vi "Keithley 6514 Buffer Config.vi"(0 "Resource In":refnum<visa-resource-name>, 1 "Check For SCPI Errors? (T)":bool=TRUE, 5 "Buffer Setup (Clear Buffer:0)":u16(ring) items=["Clear Buffer", "Configure Buffer"], 7 "Buffer Control (Never:0)":u16(ring) items=["Never", "Next"], 9 "Buffer Points (100)":i16=100 min=1 max=2500 step=1, 11 "error in (no error)":T1, 12 "TimeStamp Format (Absolute:0)":u16(ring) items=["Absolute", "Delta"], 13 "Reading Source\nfor Buffer (Sense (input):0)":u16(ring) items=["Sense (input)", "Calc1 (math)", "Calc2 (limits)"]) -> (4 "Resource Out (dupl)":refnum<visa-resource-name>, 15 "error out":T1)   [LabVIEW 2009, in "Keithley 6514 LV 2009.lvlib"]
doc: "This VI is used to configure the buffer for storing readings.\n\nDEFAULTS: GPIB Address = 14\n\nBuffer Setup:\n0 = Clear Buffer\n1 = Configure Buffer\n\nBuffer Control:\n0 = Never\n1 = Next\n\nBuffer Points:\n1 - 2500\n\nTimestamp Format:\n0 = Absolute\n1 = Delta\n\nReading source for Buffer:\n0 = Sense (input signals)\n1 = Calc1 (math)\n2 = Calc2 (limits)"
uses:
  Keithley 6514 LV 2009.lvlib
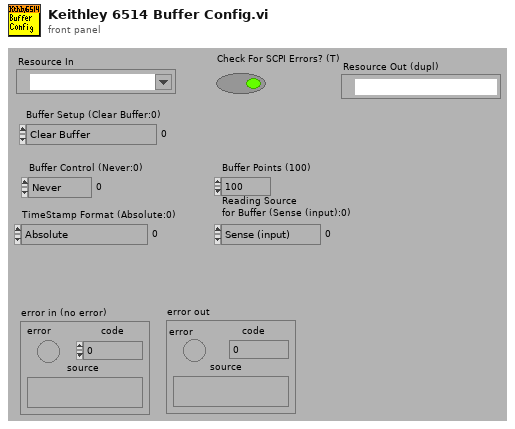
[diagram p1: front panel]
types:
  T1 = cluster{"error":bool, "code":i32, "source":string}
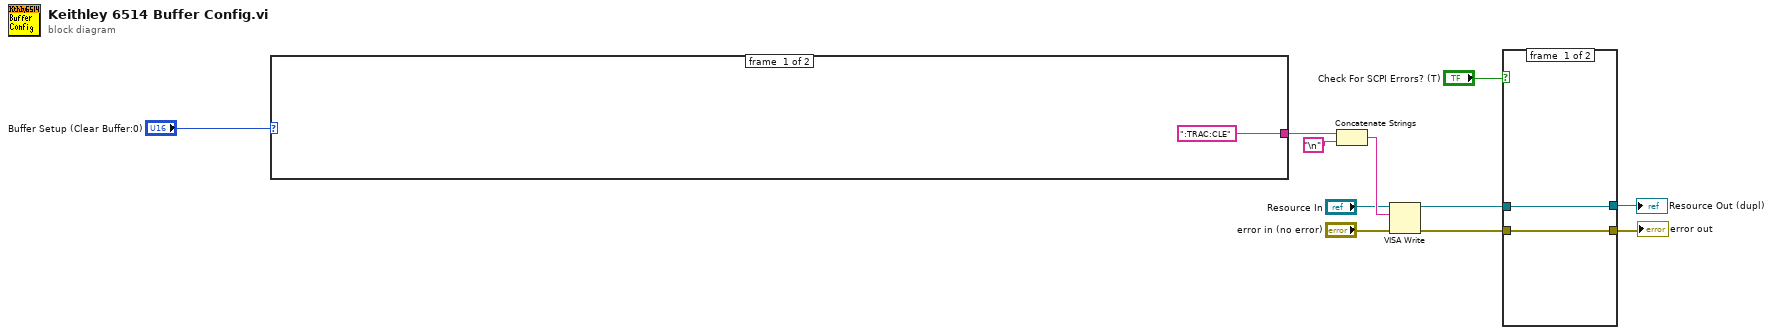
[diagram p0: block diagram]
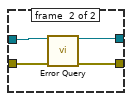
[diagram p2: hidden frame]
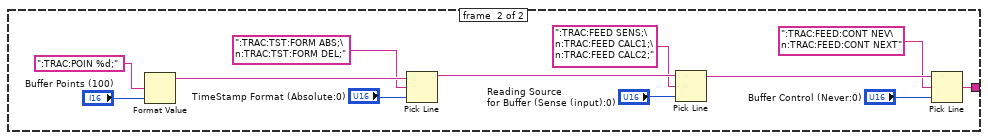
[diagram p3: hidden frame]
diagram:
  n1 = case shown="1" "Buffer Setup (Clear Buffer:0)" {
    tunnel: [":TRAC:CLE" w19] -> w10
    frame #0 {
    }
    frame #1 {
      n2 = Format Value(format string=":TRAC:POIN %d;", value (0)="Buffer Points (100)") -> (output string=w20:string)  [unwired: 1 in]
      n3 = Pick Line(string ("")=w20, multi-line string=":TRAC:TST:FORM ABS;\n:TRAC:TST:FORM DEL;", line index="TimeStamp Format (Absolute:0)") -> (output string=w17:string)
      n4 = Pick Line(string ("")=w17, multi-line string=":TRAC:FEED SENS;\n:TRAC:FEED CALC1;\n:TRAC:FEED CALC2;", line index="Reading Source\nfor Buffer (Sense (input):0)") -> (output string=w16:string)
      n5 = Pick Line(string ("")=w16, multi-line string=":TRAC:FEED:CONT NEV\n:TRAC:FEED:CONT NEXT", line index="Buffer Control (Never:0)") -> (output string=w19:string)
    }
  }
  n6 = Concatenate Strings(w10, "\n") -> (w8:string)
  n7 = VISA Write(VISA resource name="Resource In", write buffer=w8, error in (no error)="error in (no error)") -> (VISA resource name out=w4:refnum<visa-resource-name>, error out=w3:errorcluster)  [unwired: 1 out]
  n8 = case shown="False" "Check For SCPI Errors? (T)" {
    tunnel: w4 -> [w26 w30]
    tunnel: w3 -> [w25 w29]
    tunnel: [w26 w28] -> w2
    tunnel: [w25 w27] -> w1
    frame #0 {
    }
    frame #1 {
      n9 = call "Error Query.vi"("VISA Resource In"=w30, "error in (no error)"=w29) -> ("VISA Resource Out (dupl)"=w28:refnum<visa-resource-name>, "error out"=w27:errorcluster)  [unwired: 10 in, 2 out]
    }
  }
  "error out" <- w1
  "Resource Out (dupl)" <- w2
